vi "FT_Get_Latency_Timer.vi"(0 "Handle":u32) -> (1 "FT_Status":u32, 2 "Latency Timer Value":u8)   [LabVIEW 2011]
uses:
  FTD2XX.dll
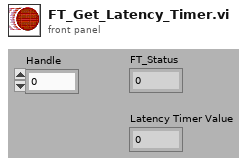
[diagram p1: front panel]
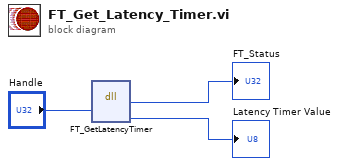
[diagram p0: block diagram]
diagram:
  n1 = dll-call lib="FTD2XX.dll" fn="FT_GetLatencyTimer"("Handle"="Handle") -> ("FT_Status"=→"FT_Status":u32, "Timer"=→"Latency Timer Value":u8)  [unwired: 4 in, 3 out]
